vi "SimpleProgram_LUM.vi"   [LabVIEW 2018, in "LumencorDLL32.lvlib"]
uses:
  LumencorDLL32.lvlib
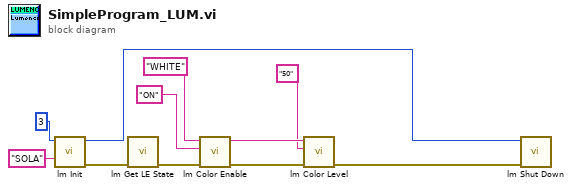
[diagram p0: block diagram]
diagram:
  n1 = call "lm Init.vi"("LETypeStr"="SOLA", "ComPort"=3) -> ("error out"=w11:errorcluster, "function return"=w5:u32)  [unwired: 7 in, 1 out]
  n2 = call "lm Get LE State.vi"("error in (no error)"=w11) -> ("error out"=w8:errorcluster)  [unwired: 9 in, 1 out]
  n3 = call "lm Color Enable.vi"("error in (no error)"=w8, "str_State"="ON", "str_Color"="WHITE") -> ("error out"=w7:errorcluster, "str_Color out"=w2:string)  [unwired: 6 in, 1 out]
  n4 = call "lm Color Level.vi"("error in (no error)"=w7, "str_Level"="50", "str_Color"=w2) -> ("error out"=w6:errorcluster)  [unwired: 6 in, 2 out]
  n5 = call "lm Shut Down.vi"("error in (no error)"=w6, "hSerial"=w5) -> ()  [unwired: 8 in, 2 out]
